vi "TPNT_CheckInRange.vi"(5 "tpnt_logfile":path, 6 "mailserver":string="localhost", 7 "check alarms":bool, 8 "error in (no error)":errorcluster, 9 "index in":i32, 10 "testpoint In":T1={"name"="", "type"="", "algor"=[], "update_rate"=0.0, "Limits"={"Alarm Type"="", "Lower "=0.0, "Upper"=0.0, "Nominal"=0.0, "outrange"=FALSE, "Check"=TRUE, "latch"=FALSE, "level"=""}, "Samples"={"samples"=0, "counter"=0, "Values"=[], "Current Value"="", "filter"="", "precision"=2}, "next_update"=0, "Status"="", "monitor"=TRUE, "error"=FALSE, "Log"={"log"=FALSE, "file"=path "", "type"="", "format"="", "updaterate"=0.0, "nex_update"=0, "mode"=""}, "permissions"="", "ID"=""} {"Log"."updaterate" format="%.2f"; "Samples"."Values" format="%.2f"; "Samples"."samples" min=1 step=1; "Limits"."Nominal" format="%.2f"; "Limits"."Upper" format="%.2f"; "Limits"."Lower" format="%.2f"; "update_rate" format="%.2f"}, 11 "device":string) -> (0 "error out":errorcluster, 2 "testpoint Out":T1={"name"="", "type"="", "algor"=[], "update_rate"=0.0, "Limits"={"Alarm Type"="", "Lower "=0.0, "Upper"=0.0, "Nominal"=0.0, "outrange"=FALSE, "Check"=TRUE, "latch"=FALSE, "level"=""}, "Samples"={"samples"=0, "counter"=0, "Values"=[], "Current Value"="", "filter"="", "precision"=2}, "next_update"=0, "Status"="", "monitor"=TRUE, "error"=FALSE, "Log"={"log"=FALSE, "file"=path "", "type"="", "format"="", "updaterate"=0.0, "nex_update"=0, "mode"=""}, "permissions"="", "ID"=""} {"Log"."updaterate" format="%.2f"; "Samples"."Values" format="%.2f"; "Samples"."samples" min=1 step=1; "Limits"."Nominal" format="%.2f"; "Limits"."Upper" format="%.2f"; "Limits"."Lower" format="%.2f"; "update_rate" format="%.2f"})   [LabVIEW 2016]
uses:
  TPNT_TP.ctl
  TPNT_Limits.ctl
  TPNT_Samples.ctl
  TPNT_Log.ctl
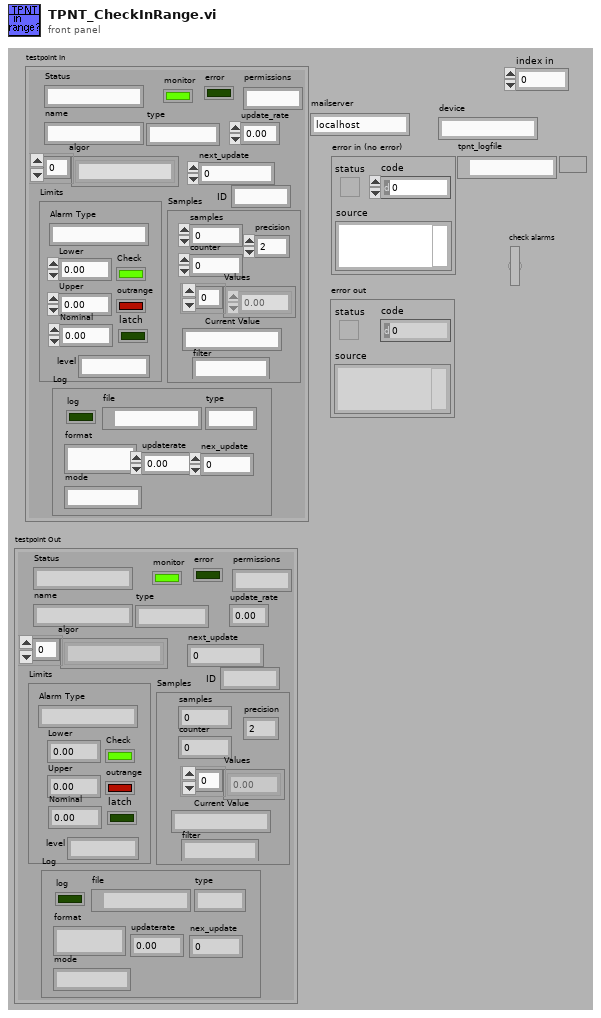
[diagram p1: front panel]
types:
  T1 = typedef "TPNT_TP.ctl" = cluster{"name":string, "type":string, "algor":string[], "update_rate":sgl, "Limits":T2, "Samples":T3, "next_update":u32, "Status":string, "monitor":bool, "error":bool, "Log":T4, "permissions":string, "ID":string}
  T2 = typedef "TPNT_Limits.ctl" = cluster{"Alarm Type":string, "Lower ":dbl, "Upper":dbl, "Nominal":dbl, "outrange":bool, "Check":bool, "latch":bool, "level":string}
  T3 = typedef "TPNT_Samples.ctl" = cluster{"samples":i32, "counter":i32, "Values":dbl[], "Current Value":string, "filter":string, "precision":u8}
  T4 = typedef "TPNT_Log.ctl" = cluster{"log":bool, "file":path, "type":string, "format":string, "updaterate":dbl, "nex_update":u32, "mode":string}
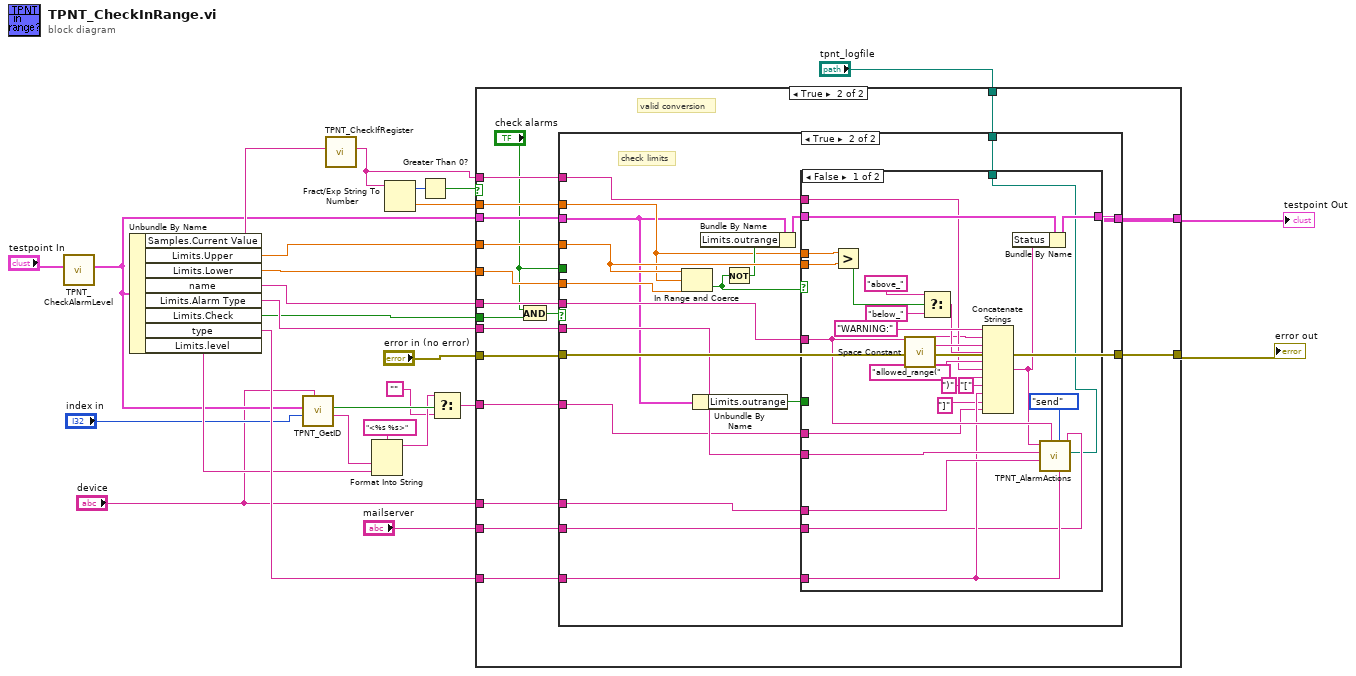
[diagram p0: block diagram]
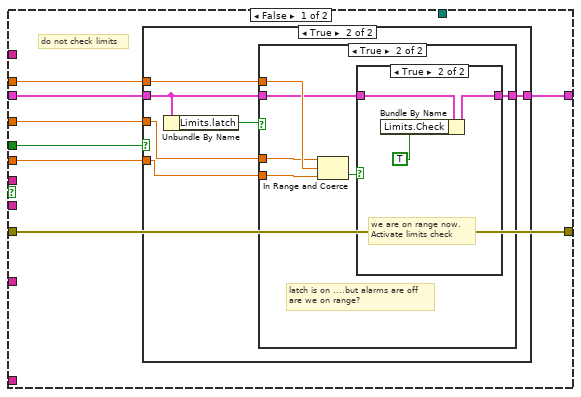
[diagram p3: hidden frame]
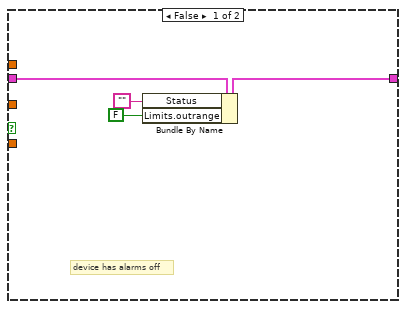
[diagram p4: hidden frame]
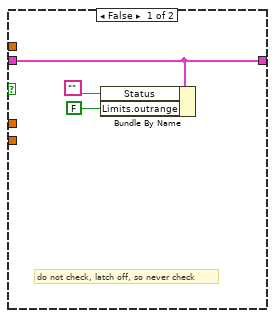
[diagram p5: hidden frame]
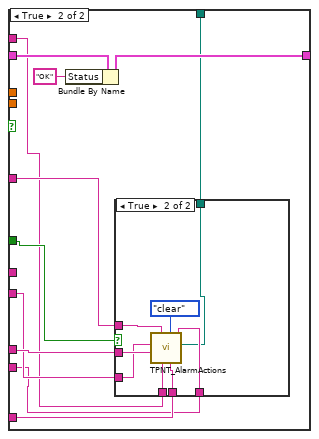
[diagram p7: hidden frame]
diagram:
  n1 = call "TPNT_CheckAlarmLevel.vi"("testpoint In"="testpoint In") -> ("testpoint out"=w7:T1)  [unwired: 10 out]
  n2 = Unbundle By Name(w7) -> ("Samples.Current Value"=w15:string, "Limits.Upper"=w24:dbl, "Limits.Lower"=w23:dbl, "name"=w22:string, "Limits.Alarm Type"=w21:string, "Limits.Check"=w20:bool, "type"=w16:string, "Limits.level"=w11:string)
  n3 = call "TPNT_GetID.vi"("device"="device", "index in"="index in", "testpoint In"=w7) -> ("id out"=w5:string, "id?"=w6:bool)  [unwired: 7 out]
  n4 = call "TPNT_CheckIfRegister.vi"("value in"=w15) -> ("value out"=w14:string)  [unwired: 10 out]
  n5 = Format Into String(format string="<%s %s>", w5, w11) -> (resulting string=w3:string)  [unwired: 2 in, 1 out]
  n6 = Fract/Exp String To Number(string=w14) -> (offset past number=w18:i32, number=w19:dbl)  [unwired: 3 out]
  n7 = Greater Than 0?(x=w18) -> (x > 0?=w17:bool)
  n8 = Select(t=w3, s=w6, f="") -> (s? t:f=w10:string)
  n9 = case shown="True" w17 {
    tunnel: w7 -> [w29 w47]
    tunnel: [w29 w46] -> w27
    tunnel: "error in (no error)" -> [w28 w45]
    tunnel: [w28 w44] -> w25
    tunnel: w24 -> [_ w43]
    tunnel: w23 -> [_ w42]
    tunnel: w22 -> [_ w41]
    tunnel: w21 -> [_ w40]
    tunnel: w20 -> [_ w39]
    tunnel: w14 -> [_ w37]
    tunnel: w19 -> [_ w36]
    tunnel: w16 -> [_ w34]
    tunnel: "mailserver" -> [_ w33]
    tunnel: w10 -> [_ w32]
    tunnel: "tpnt_logfile" -> [_ w31]
    tunnel: "device" -> [_ w30]
    frame False {
      # "wrong conversion. It may be an ascii message. Pass it through"
    }
    frame True {
      # "valid conversion"
      n10 = And(x="check alarms", y=w39) -> (x .and. y?=w38:bool)
      n11 = case shown="True" w38 {
        tunnel: w47 -> [w53 w84]
        tunnel: [w52 w92] -> w46
        tunnel: w45 -> [w54 w91]
        tunnel: [w54 w91] -> w44
        tunnel: w43 -> [w49 w90]
        tunnel: w42 -> [w48 w95]
        tunnel: w41 -> [_ w89]
        tunnel: w40 -> [_ w85]
        tunnel: w37 -> [_ w87]
        tunnel: w36 -> [w50 w86]
        tunnel: "check alarms" -> [w51 _]
        tunnel: w34 -> [_ w82]
        tunnel: w33 -> [_ w81]
        tunnel: w32 -> [_ w80]
        tunnel: w31 -> [_ w79]
        tunnel: w30 -> [_ w78]
        frame False {
          # "do not check limits"
          n12 = case shown="True" w51 {
            tunnel: w53 -> [w58 w63]
            tunnel: [w57 w62] -> w52
            tunnel: w50 -> [_ w61]
            tunnel: w49 -> [_ w60]
            tunnel: w48 -> [_ w59]
            frame False {
              # "device has alarms off"
              n13 = Bundle By Name(cluster=w58, "Status"="", "Limits.outrange"=FALSE) -> (w57:T1)
            }
            frame True {
              n14 = Unbundle By Name(w63) -> ("Limits.latch"=w64:bool)
              n15 = case shown="True" w64 {
                tunnel: w63 -> [w67 w69]
                tunnel: [w67 w68] -> w62
                tunnel: w61 -> [_ w73]
                tunnel: w60 -> [_ w72]
                tunnel: w59 -> [_ w71]
                frame False {
                  # "do not check, latch off, so never check"
                  n16 = Bundle By Name(cluster=w67, "Status"="", "Limits.outrange"=FALSE) -> ()  [unwired: 1 out]
                }
                frame True {
                  # "latch is on ....but alarms are off\nare we on range?"
                  n17 = In Range and Coerce(upper limit=w72, x=w73, lower limit=w71) -> (In Range?=w70:bool)  [unwired: 1 out]
                  n18 = case shown="True" w70 {
                    tunnel: w69 -> [w74 w77]
                    tunnel: [w74 w75] -> w68
                    frame False {
                      # "still out of range\ndo not activate limits check"
                    }
                    frame True {
                      # "we are on range now.\nActivate limits check"
                      n19 = Bundle By Name(cluster=w77, "Limits.Check"=TRUE) -> (w75:T1)
                    }
                  }
                }
              }
            }
          }
        }
        frame True {
          # "check limits"
          n20 = In Range and Coerce(upper limit=w90, x=w86, lower limit=w95) -> (In Range?=w94:bool)  [unwired: 1 out]
          n21 = Unbundle By Name(w84) -> ("Limits.outrange"=w83:bool)
          n22 = Not(x=w94) -> (.not. x?=w88:bool)
          n23 = Bundle By Name(cluster=w84, "Limits.outrange"=w88) -> (w93:T1)
          n24 = case shown="False" w94 {
            tunnel: w93 -> [w119 w130]
            tunnel: [w118 w128] -> w92
            tunnel: w86 -> [w117 _]
            tunnel: w90 -> [w116 _]
            tunnel: w89 -> [w105 w125]
            tunnel: w87 -> [w108 w123]
            tunnel: w85 -> [w106 w124]
            tunnel: w83 -> [_ w127]
            tunnel: w78 -> [w104 w126]
            tunnel: w82 -> [w101 w122]
            tunnel: w81 -> [w99 w121]
            tunnel: w80 -> [w98 _]
            tunnel: w79 -> [w96 w120]
            frame False {
              n25 = Greater?(x=w117, y=w116) -> (0:w115:bool)
              n26 = call <vilib>:"Space Constant.vi"() -> ("String"=w111:string)
              n27 = Select(t="above_", s=w115, f="below_") -> (s? t:f=w110:string)
              n28 = Concatenate Strings("WARNING:", w105, w111, w110, "allowed_range(" ("string"), w108, ")" ("string"), "[" ("string"), w101, "]" ("string"), w98) -> (w97:string)
              n29 = Bundle By Name(cluster=w119, "Status"=w97) -> (w118:T1)
              n30 = call "TPNT_AlarmActions.vi"("tpnt_logfile"=w96, "mailserver"=w99, "tpnt type"=w101, "action"=enum16{"send", "clear", "clear all"}."send", "TP name"=w105, "device"=w104, "alarm field"=w106, "alarm message"=w97) -> ()  [unwired: 2 in, 2 out]
            }
            frame True {
              n31 = Bundle By Name(cluster=w130, "Status"="OK") -> (w128:T1)
              n32 = case shown="True" w127 {
                tunnel: w126 -> [_ w138]
                tunnel: w125 -> [_ w137]
                tunnel: w124 -> [_ w136]
                tunnel: w123 -> [_ w135]
                tunnel: w122 -> [_ w133]
                tunnel: w121 -> [_ w132]
                tunnel: w120 -> [_ w131]
                frame False {
                }
                frame True {
                  n33 = call "TPNT_AlarmActions.vi"("tpnt_logfile"=w131, "mailserver"=w132, "tpnt type"=w133, "action"=enum16{"send", "clear", "clear all"}."clear", "curr val"=w135, "TP name"=w137, "device"=w138, "alarm field"=w136) -> ()  [unwired: 2 in, 2 out]
                }
              }
            }
          }
        }
      }
    }
  }
  "error out" <- w25
  "testpoint Out" <- w27
